vi "MicroStruct-Dots.vi"() -> ()   [LabVIEW 2014]
doc: "Newport Motion Controler\nThis program make lines structure\n\nAndré Romero - 2020\nandretec@ifsc.usp.br"
uses:
  <vilib>/Platform/TimedLoop/XDataNode/wakeup.ctl
  <vilib>/Platform/TimedLoop/XDataNode/XDNodeRunTimeDep.lvlib
  <vilib>/Platform/TimedLoop/XDataNode/nitl_modes.ctl
  <vilib>/Platform/TimedLoop/XDataNode/timing_clust.ctl
  <vilib>/Platform/TimedLoop/XDataNode/XDataNode.xnode
  Basic-VIs/Global Motor Axis.vi
panel:
  in  "Dots layout":u16(ring) items=["Layout 1", "Layout 2"]
  out "Space bet dots (mm)":dbl
  in  "GO":bool
  in  "Time Dots (ms)":u32=1000 min=1
  in  "N Dots / L":i32=5 min=1
  in  "Swap motor":bool
  out "XY Graph":cluster{dbl[], dbl[]}(graph)={[0.0, 0.0, 0.0345, 0.108, 0.2205, 0.3735, 0.564, 0.7665, 0.964, 1.0005, 1.0, 0.9995, 0.9995, 0.9815, 0.9225, 0.8235, 0.686, 0.505, 0.308, 0.108, -0.002, 0.0, 0.0005, 0.0, 0.012, 0.066, 0.1575, 0.2915, 0.465, 0.6645, 0.866, 1.0025, 1.0, 1.0, 0.9995, 0.9965, 0.9565, 0.8775, 0.7585, 0.6, 0.4055, 0.204, 0.006, -0.0005, 0.0005, 0.0, 0.0005, 0.0345, 0.108, 0.2215, 0.375, 0.566, 0.7675, 0.9685, 1.001, 1.0, 1.0, 0.9995, 0.9855, 0.9315, 0.8375, 0.7035, 0.5295, 0.331, 0.1305, -0.0025, 0.0, 0.0005, 0.0, 0.009, 0.0585, 0.148, 0.2765, 0.4475, 0.645, 0.8435, 1.003, 1.0005, 1.0, 0.9995, 0.999, 0.9625, 0.887, 0.773, 0.6175, 0.4265, 0.225, 0.028, -0.0005, 0.0005, 0.0, 0.0005, 0.031, 0.1025, 0.2125, 0.364, 0.55, 0.751, 0.9525, 1.001, 1.0, 1.0, 0.9995, 0.986, 0.9315, 0.8385, 0.705, 0.531, 0.3315, 0.1305, -0.002, 0.0, 0.0005, 0.0, 0.0085, 0.057, 0.146, 0.2735, 0.44, 0.6395, 0.8415, 1.003, 1.0, 1.0, 1.0, 0.9995, 0.9645, 0.891, 0.7775, 0.6255, 0.4355, 0.2345, 0.033, -0.0005, 0.0005, 0.0, 0.0, 0.0185, 0.0775, 0.1765, 0.3145, 0.4925, 0.6925, 0.895, 1.002, 1.0, 1.0, 0.9995, 0.9865, 0.933, 0.839, 0.7055, 0.535, 0.333, 0.1325, -0.0025, 0.0, 0.0005, 0.0, 0.0025, 0.043, 0.1225, 0.2425, 0.4015, 0.5945, 0.795, 0.9955, 1.0005, 1.0, 1.0, 0.9995, 0.965, 0.8915, 0.7775, 0.625, 0.4335, 0.235, 0.035, -0.0005, 0.0005, 0.0, 0.0, 0.0185, 0.078, 0.176, 0.3155, 0.4925, 0.693, 0.892, 1.002, 1.0, 1.0, 0.9995, 0.9865, 0.933, 0.8405, 0.706, 0.5345, 0.3325, 0.1335, -0.0025, 0.0, 0.0005, 0.0, 0.002, 0.043, 0.1225, 0.2415, 0.401, 0.594, 0.7955, 0.9945, 1.0005, 1.0, 0.9995, 0.9995, 0.9655, 0.891, 0.7775, 0.623, 0.431, 0.233, 0.032, 0.0, 0.0005, 0.0, 0.0], [0.0, 0.0, 0.0, 0.0, 0.0, 0.0, 0.0, 0.0, 0.0, 0.0, 0.021, 0.0825, 0.1015, 0.101, 0.1005, 0.1, 0.1, 0.1, 0.1, 0.1, 0.1, 0.104, 0.158, 0.2015, 0.2015, 0.2005, 0.2, 0.2, 0.2, 0.2, 0.2, 0.2, 0.2, 0.2425, 0.3015, 0.3015, 0.301, 0.3005, 0.3, 0.3, 0.3, 0.3, 0.3, 0.3, 0.328, 0.3975, 0.4015, 0.401, 0.4005, 0.4, 0.4, 0.4, 0.4, 0.4, 0.4, 0.411, 0.468, 0.5015, 0.501, 0.5005, 0.5, 0.5, 0.5, 0.5, 0.5, 0.5, 0.504, 0.557, 0.6015, 0.601, 0.6005, 0.6, 0.6, 0.6, 0.6, 0.6, 0.6, 0.6, 0.6365, 0.7015, 0.7015, 0.701, 0.7, 0.7, 0.7, 0.7, 0.7, 0.7, 0.7, 0.7275, 0.7955, 0.8015, 0.801, 0.8005, 0.8, 0.8, 0.8, 0.8, 0.8, 0.8, 0.8105, 0.868, 0.902, 0.9015, 0.9, 0.9, 0.9, 0.9, 0.9, 0.9, 0.9, 0.9005, 0.9485, 1.0015, 1.0015, 1.0005, 1.0, 1.0, 1.0, 0.9995, 0.9995, 1.0, 1.0, 1.0345, 1.1015, 1.1015, 1.101, 1.1, 1.1, 1.1, 1.1, 1.1, 1.1, 1.1, 1.128, 1.1865, 1.2015, 1.201, 1.2, 1.2, 1.2, 1.1995, 1.2, 1.2, 1.2, 1.207, 1.259, 1.3015, 1.3015, 1.3005, 1.3, 1.3, 1.3, 1.3, 1.3, 1.3, 1.3, 1.343, 1.4015, 1.4015, 1.4005, 1.4, 1.4, 1.4, 1.4, 1.3995, 1.3995, 1.4, 1.429, 1.4985, 1.5015, 1.5005, 1.5, 1.5, 1.5, 1.5, 1.5, 1.5, 1.5, 1.5175, 1.578, 1.6015, 1.601, 1.6005, 1.6, 1.6, 1.6, 1.6, 1.6, 1.6, 1.605, 1.659, 1.7015, 1.701, 1.7005, 1.7, 1.7, 1.7, 1.7, 1.7, 1.7, 1.7, 1.7425, 1.802, 1.8015, 1.8005, 1.8, 1.8, 1.8, 1.8, 1.8, 1.8, 1.8, 1.8295, 1.8995, 1.9015, 1.9005, 1.9, 1.9, 1.9, 1.9, 1.9, 1.8995, 1.8995, 1.918, 1.979, 2.002]}
  in  "N Cycles":i32=10 min=1
  in  "Acceleration (0 units/s²)":dbl=1.0 min=0.0 format="%#.4g"
  in  "Velocity (units/s)":dbl=1.0 min=0.0 format="%#.4g"
  in  "d (mm)":dbl=10.0
  in  "L (mm)":dbl=1.0
  out "X Position (mm)":dbl format="%.6g"
  out "Y Position (mm)":dbl=2.002 format="%.6g"
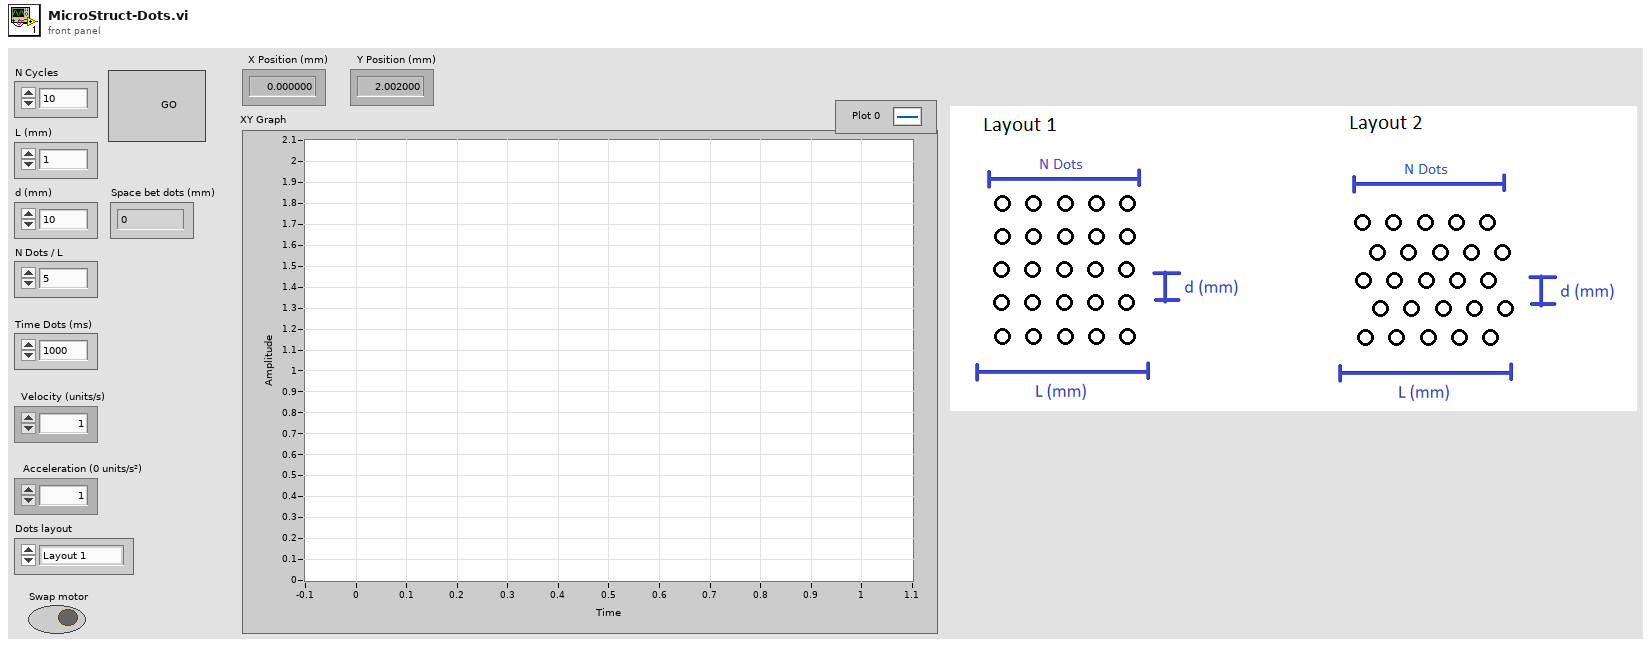
[diagram p1: front panel]
types:
  T1 = typedef "XDNodeRunTimeDep.lvlib/timing_clust.ctl" = cluster{"Expected End [f-1]":u64, "Actual End [f-1]":u64, "Finished Late? [f-1]":bool, "Expected End [i-1]":u64, "Actual End [i-1]":u64, "Finished Late? [i-1]":bool, "Expected Start [i]":u64, "Actual Start [i]":u64, "Expected Start [f]":u64, "Actual Start [f]":u64, "Source Name":string, "Structure Name":string, "Period":i64, "Deadline":i64, "Offset":i64, "Start":i64, "Priority":i32, "Timeout":i32, "Mode":T2, "Wakeup Reason":T3, "Error":errorcluster, "Source Type":string, "Secondary Source Type":string, "Global End Time":u64, "Global Start Time":u64, "Frame Duration":u64, "Iteration Duration":u64, "Assigned CPU":i32, "I/O Scan Engine Mode":u32}
  T2 = typedef "XDNodeRunTimeDep.lvlib/nitl_modes.ctl" = enum32{"No Change", "Process missed periods, maintain original phase", "Discard missed periods, maintain original phase", "Process missed periods, ignore original phase", "Discard missed periods, ignore original phase"}
  T3 = typedef "XDNodeRunTimeDep.lvlib/wakeup.ctl" = enum32{"Normal", "Aborted", "Asynchronous wakeup", "Timing source error", "Timed loop error", "Timeout"}
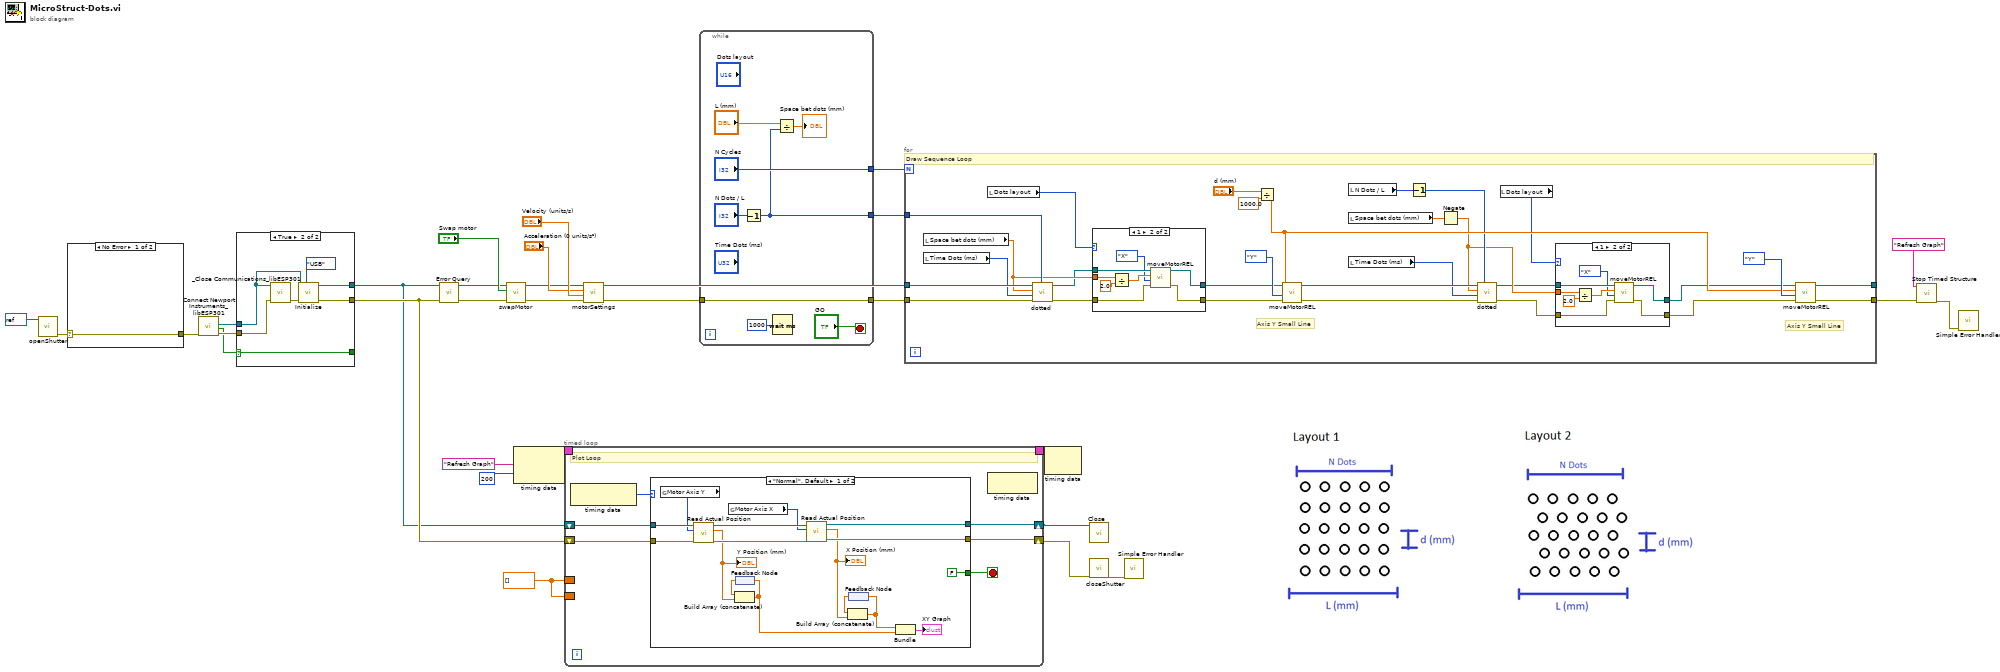
[diagram p0: block diagram]
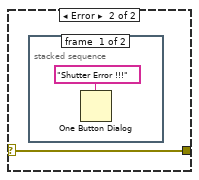
[diagram p2: hidden frame]
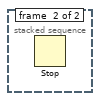
[diagram p3: hidden frame]
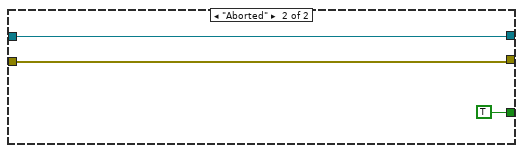
[diagram p6: hidden frame]
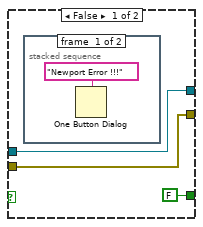
[diagram p7: hidden frame]
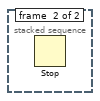
[diagram p8: hidden frame]
diagram:
  w17 = dbl[] []
  n1 = call "openShutter.vi"("VISA Refnum in"=refnum<visa-resource-name> refnum) -> ("error out"=w8:errorcluster)  [unwired: 9 in, 1 out]
  n2 = case shown="No Error" w8 {
    selector: w8 -> [w32 w33]
    tunnel: [w32 w33] -> w7
    frame No Error {
    }
    frame Error {
      n3 = stacked-sequence {
        frame #0 {
          n4 = One Button Dialog(message="Shutter Error !!!") -> ()  [unwired: 1 in, 1 out]
        }
        frame #1 {
          n5 = Stop() -> ()  [unwired: 1 in]
        }
      }
    }
  }
  n6 = call <userlib>:"Connect Newport Instruments_libESP301.vi"("error in (no error)"=w7) -> ("error (duplicate)"=w31:errorcluster, "Connected"=w26:bool, "VISA resource name (duplicate)"=w30:refnum<visa-resource-name>)  [unwired: 6 in, 2 out]
  n7 = case shown="True" w26 {
    selector: w26 -> [_ w39]
    tunnel: w31 -> [w35 w43]
    tunnel: w30 -> [w36 w42]
    tunnel: [w35 w41] -> w29
    tunnel: [w36 w40] -> w28
    tunnel: [FALSE w39] -> _
    frame False {
      n8 = stacked-sequence {
        frame #0 {
          n9 = One Button Dialog(message="Newport Error !!!") -> ()  [unwired: 1 in, 1 out]
        }
        frame #1 {
          n10 = Stop() -> ()  [unwired: 1 in]
        }
      }
    }
    frame True {
      n11 = call <userlib>:"_Close Communications_libESP301.vi"("Instrument Channel"=w42, "error in (no error)"=w43) -> ("error out"=w45:errorcluster)  [unwired: 13 in]
      n12 = call <userlib>:"Initialize.vi"("VISA resource name"=w42, "error in (no error)"=w45, "Serial Link (RS232)"=enum16{"RS232", "USB"}."USB") -> ("VISA resource name out"=w40:refnum<visa-resource-name>, "error out"=w41:errorcluster)  [unwired: 6 in]
    }
  }
  n13 = call <userlib>:"Error Query.vi"("error in (no error)"=w29, "VISA resource name"=w28) -> ("error out"=w12:errorcluster, "VISA resource name out"=w13:refnum<visa-resource-name>)  [unwired: 2 in, 2 out]
  n14 = call "swapMotor.vi"("error in (no error)"=w12, "Swap motor"="Swap motor", "VISA Refnum in"=w13) -> ("error out"=w10:errorcluster, "VISA Refnum out"=w11:refnum<visa-resource-name>)  [unwired: 7 in]
  n15 = node-c288("Refresh Graph" ("Structure Name"), i64 200 ("Period")) -> (w25:T1)
  n16 = timed-loop {
    timing: w25 -> [_]
    timing-out: [_] -> w24
    shift-right: [w49] -> w27
    shift-left: w28 -> [w51]
    shift-right: [w48] -> w2
    shift-left: w29 -> [w50]
    border: w17 -> [_]
    border: w17 -> [_]
    stop <- w46 stop-if-true
    # "Plot Loop"
    n17 = node-c288() -> (w47:T3)  [unwired: 1 in]
    n18 = case shown="\"Normal\", Default" w47 {
      tunnel: w51 -> [w67 w69]
      tunnel: w50 -> [w66 w68]
      tunnel: [w63 w69] -> w49
      tunnel: [w62 w68] -> w48
      tunnel: [FALSE TRUE] -> w46
      frame "Normal", Default {
        n19 = global read "Global Motor Axis.vi" "Motor Axis Y"() -> (w52:i32)
        n20 = call <userlib>:"Read Actual Position.vi"("error in (no error)"=w66, "Axis (1)"=w52, "VISA resource name"=w67) -> ("error out"=w64:errorcluster, "Position (units)"=w57:dbl, "VISA resource name out"=w65:refnum<visa-resource-name>)  [unwired: 2 in]
        "Y Position (mm)" <- w57
        n21 = global read "Global Motor Axis.vi" "Motor Axis X"() -> (w53:i32)
        n22 = feedback #1() -> (w60:dbl[])
        n23 = Build Array (concatenate)(w60, w57) -> (w55:dbl[])
        n24 = feedback-in #1(w55) -> ()
        n25 = call <userlib>:"Read Actual Position.vi"("error in (no error)"=w64, "Axis (1)"=w53, "VISA resource name"=w65) -> ("error out"=w62:errorcluster, "Position (units)"=w58:dbl, "VISA resource name out"=w63:refnum<visa-resource-name>)  [unwired: 2 in]
        "X Position (mm)" <- w58
        n26 = feedback #2() -> (w59:dbl[])
        n27 = Build Array (concatenate)(w59, w58) -> (w56:dbl[])
        n28 = feedback-in #2(w56) -> ()
        n29 = Bundle(w56, w55) -> (→"XY Graph":cluster{dbl[], dbl[]})  [unwired: 1 in]
      }
      frame "Aborted" {
      }
    }
    n30 = node-c288() -> ()  [unwired: 1 in, 1 out]
  }
  n31 = call "motorSettings.vi"("error in (no error)"=w10, "Velocity (units/s)"="Velocity (units/s)", "Acceleration (0 units/s²)"="Acceleration (0 units/s²)", "VISA Refnum in"=w11) -> ("error out"=w6:errorcluster, "VISA Refnum out"=w20:refnum<visa-resource-name>)  [unwired: 6 in]
  n32 = while {
    tunnel: w6 -> [w81]
    tunnel: [w81] -> w5
    tunnel: ["N Cycles"] -> w4
    tunnel: [w74] -> w3
    stop <- "GO" stop-if-true
    n33 = Decrement(x="N Dots / L") -> (x-1=w74:i32)
    n34 = Wait (ms)(milliseconds to wait=u32 1000) -> ()  [unwired: 1 out]
    n35 = Divide(x="L (mm)", y=w74) -> (x/y=→"Space bet dots (mm)":dbl)
  }
  n36 = for {
    N: w4 -> [_]
    tunnel: w20 -> [w103]
    tunnel: w5 -> [w102]
    tunnel: [w107] -> _
    tunnel: [w106] -> w16
    tunnel: w3 -> [w101]
    # "Axis Y Small Line"
    # "Axis Y Small Line"
    # "Draw Sequence Loop"
    n37 = local read "Space bet dots (mm)"() -> (w90:dbl)
    n38 = local read "Time Dots (ms)"() -> (w99:u32)
    n39 = local read "Dots layout"() -> (w93:u16)
    n40 = call "dotted.vi"("N times"=w101, "error in (no error)"=w102, "Time Dots (ms)"=w99, "Space bet dots (mm)"=w90, "VISA Refnum in"=w103) -> ("error out"=w92:errorcluster, "VISA Refnum out"=w89:refnum<visa-resource-name>)  [unwired: 5 in]
    n41 = case shown="1" w93 {
      tunnel: w92 -> [w122 w127]
      tunnel: [w122 w126] -> w91
      tunnel: w90 -> [_ w130]
      tunnel: w89 -> [w121 w125]
      tunnel: [w121 w124] -> w88
      frame 0, Default {
      }
      frame 1 {
        n42 = Divide(x=w130, y=2.0) -> (x/y=w128:dbl)
        n43 = call "moveMotorREL.vi"("error in (no error)"=w127, "Axis"=enum16{"X", "Y"}."X", "L (mm)"=w128, "VISA Refnum in"=w125) -> ("error out"=w126:errorcluster, "VISA Refnum out"=w124:refnum<visa-resource-name>)  [unwired: 6 in]
      }
    }
    n44 = Divide(x="d (mm)", y=1000.0) -> (x/y=w104:dbl)
    n45 = call "moveMotorREL.vi"("error in (no error)"=w91, "Axis"=enum16{"X", "Y"}."Y", "L (mm)"=w104, "VISA Refnum in"=w88) -> ("error out"=w97:errorcluster, "VISA Refnum out"=w98:refnum<visa-resource-name>)  [unwired: 6 in]
    n46 = local read "N Dots / L"() -> (w95:i32)
    n47 = local read "Space bet dots (mm)"() -> (w100:dbl)
    n48 = local read "Time Dots (ms)"() -> (w96:u32)
    n49 = Decrement(x=w95) -> (x-1=w94:i32)
    n50 = Negate(x=w100) -> (-x=w87:dbl)
    n51 = call "dotted.vi"("N times"=w94, "error in (no error)"=w97, "Time Dots (ms)"=w96, "Space bet dots (mm)"=w87, "VISA Refnum in"=w98) -> ("error out"=w84:errorcluster, "VISA Refnum out"=w86:refnum<visa-resource-name>)  [unwired: 5 in]
    n52 = local read "Dots layout"() -> (w85:u16)
    n53 = case shown="1" w85 {
      tunnel: w84 -> [w112 w117]
      tunnel: [w112 w116] -> w82
      tunnel: w87 -> [_ w120]
      tunnel: w86 -> [w111 w115]
      tunnel: [w111 w114] -> w83
      frame 0, Default {
      }
      frame 1 {
        n54 = Divide(x=w120, y=2.0) -> (x/y=w118:dbl)
        n55 = call "moveMotorREL.vi"("error in (no error)"=w117, "Axis"=enum16{"X", "Y"}."X", "L (mm)"=w118, "VISA Refnum in"=w115) -> ("error out"=w116:errorcluster, "VISA Refnum out"=w114:refnum<visa-resource-name>)  [unwired: 6 in]
      }
    }
    n56 = call "moveMotorREL.vi"("error in (no error)"=w82, "Axis"=enum16{"X", "Y"}."Y", "L (mm)"=w104, "VISA Refnum in"=w83) -> ("error out"=w106:errorcluster, "VISA Refnum out"=w107:refnum<visa-resource-name>)  [unwired: 6 in]
  }
  n57 = node-c288(w24) -> ()  [unwired: 1 out]
  n58 = call <userlib>:"Close.vi"("VISA resource name"=w27) -> ()  [unwired: 10 in, 1 out]
  n59 = call "closeShutter.vi"("Error In"=w2) -> ("Error Out"=w1:errorcluster)  [unwired: 10 in]
  n60 = call <vilib>:"Simple Error Handler.vi"("error in (no error)"=w1) -> ()  [unwired: 1 in, 8 out]
  n61 = call <vilib>:"Stop Timed Structure.vi"("error in (no error)"=w16, "name"="Refresh Graph" ("Structure Name")) -> ("error out"=w15:errorcluster)  [unwired: 9 in]
  n62 = call <vilib>:"Simple Error Handler.vi"("error in (no error)"=w15) -> ()  [unwired: 4 in, 5 out]
